vi "Extract Raw Data To Real Data.vi"(11 "data":u8[](array[numeric])) -> (0 "Step":u8, 1 "Communication":u8, 2 "Auto Running":bool, 3 "Test Cycle Running":bool, 4 "Fault":bool[](array[boolean]), 5 "test status":u8, 6 "DI 0-31":bool[](array[boolean]), 8 "DO 0-31 2":bool[](array[boolean]))   [LabVIEW 2015]
panel:
  out "DO 0-7":bool[](array[boolean])
  out "DO 8-15":bool[](array[boolean])
  out "DO16-23":bool[](array[boolean])
  out "DO 24-31":bool[](array[boolean])
  out "DI16-23":bool[](array[boolean])
  out "DI 24-31":bool[](array[boolean])
  out "DI 8-15":bool[](array[boolean])
  out "DI 0-7":bool[](array[boolean])
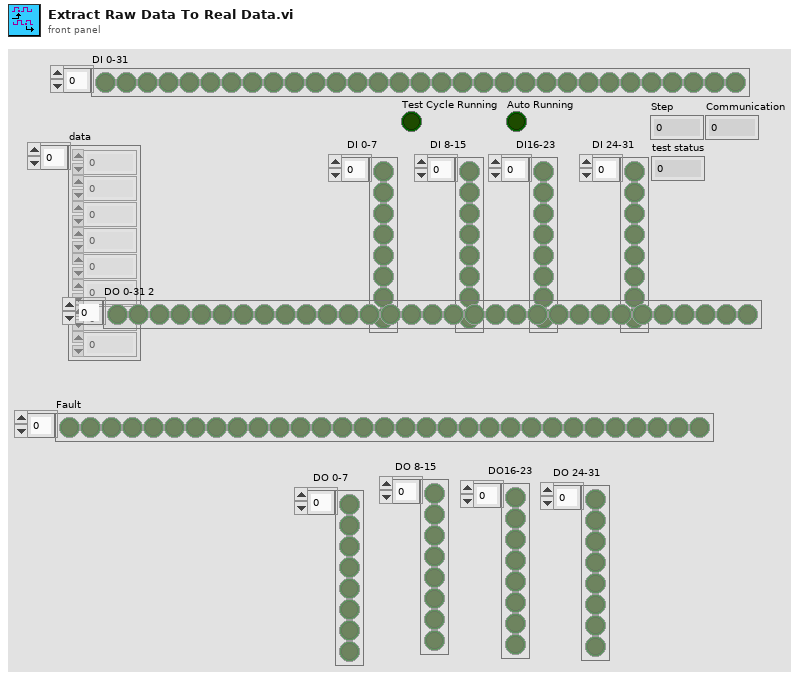
[diagram p1: front panel]
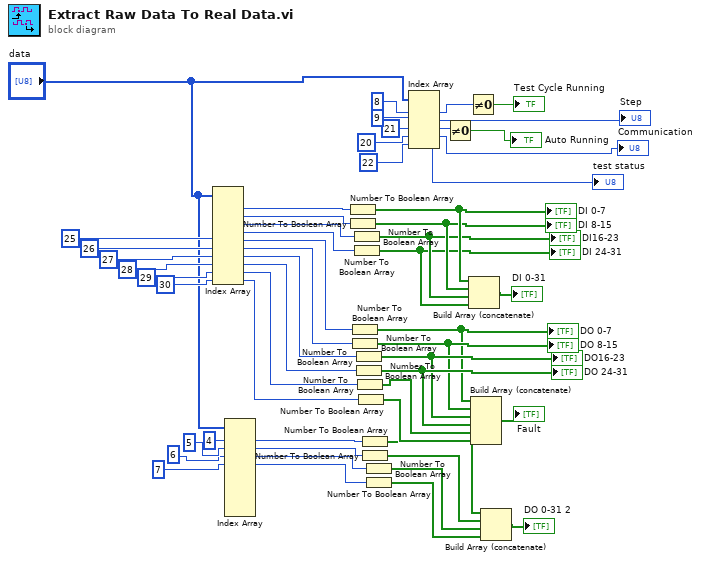
[diagram p0: block diagram]
diagram:
  n1 = Index Array(array="data", index #5=25 ("index"), index #6=26 ("index"), index #7=27 ("index"), index #8=28 ("index"), index #9=29 ("index"), index #10=30 ("index")) -> (element #1=w54:u8, element #2=w53:u8, element #3=w52:u8, element #4=w51:u8, element #5=w41:u8, element #6=w40:u8, element #7=w39:u8, element #8=w38:u8, element #9=w30:u8, element #10=w29:u8)  [unwired: 4 in]
  n2 = Index Array(array="data", index #1=4 ("index"), index #2=5 ("index"), index #3=6 ("index"), index #4=7 ("index")) -> (element #1=w8:u8, element #2=w9:u8, element #3=w10:u8, element #4=w11:u8)  [unwired: 6 in, 6 out]
  n3 = Number To Boolean Array(number=w54) -> (Boolean array=w50:bool[])
  "DI 0-7" <- w50
  n4 = Number To Boolean Array(number=w53) -> (Boolean array=w49:bool[])
  "DI 8-15" <- w49
  n5 = Number To Boolean Array(number=w41) -> (Boolean array=w42:bool[])
  "DO 0-7" <- w42
  n6 = Number To Boolean Array(number=w40) -> (Boolean array=w43:bool[])
  "DO 8-15" <- w43
  n7 = Number To Boolean Array(number=w52) -> (Boolean array=w48:bool[])
  "DI16-23" <- w48
  n8 = Number To Boolean Array(number=w51) -> (Boolean array=w47:bool[])
  "DI 24-31" <- w47
  n9 = Number To Boolean Array(number=w39) -> (Boolean array=w44:bool[])
  "DO16-23" <- w44
  n10 = Number To Boolean Array(number=w38) -> (Boolean array=w45:bool[])
  "DO 24-31" <- w45
  n11 = Number To Boolean Array(number=w30) -> (Boolean array=w28:bool[])
  n12 = Number To Boolean Array(number=w29) -> (Boolean array=w27:bool[])
  n13 = Number To Boolean Array(number=w8) -> (Boolean array=w12:bool[])
  n14 = Number To Boolean Array(number=w9) -> (Boolean array=w13:bool[])
  n15 = Number To Boolean Array(number=w10) -> (Boolean array=w14:bool[])
  n16 = Number To Boolean Array(number=w11) -> (Boolean array=w15:bool[])
  n17 = Index Array(array="data", index #1=8 ("index"), index #2=9 ("index"), index #3=21 ("index"), index #4=20 ("index"), index #5=22 ("index")) -> (element #1=w25:u8, element #2=→"Step":u8, element #3=w22:u8, element #4=→"Communication":u8, element #5=→"test status":u8)
  n18 = Not Equal To 0?(x=w22) -> (x != 0?=→"Auto Running":bool)
  n19 = Not Equal To 0?(x=w25) -> (x != 0?=→"Test Cycle Running":bool)
  n20 = Build Array (concatenate)(w50, w49, w48, w47) -> (→"DI 0-31":bool[])
  n21 = Build Array (concatenate)(w42, w43, w44, w45, w28, w27) -> (→"Fault":bool[])
  n22 = Build Array (concatenate)(w12, w13, w14, w15) -> (→"DO 0-31 2":bool[])
